vi "CheckStatusFlag.vi"(8 "error in (no error)":errorcluster, 11 "CS++Message in":refnum<class "CS++Message.lvclass">) -> (0 "error out":errorcluster, 3 "CS++Message out":refnum<class "CS++Message.lvclass">)   [LabVIEW 2016, in "CS++Message.lvlib" / "CS++Message.lvclass"]
uses:
  CS++Message.lvclass
  CS++Message.lvclass/CS++Message.ctl
  MessageStatus.ctl
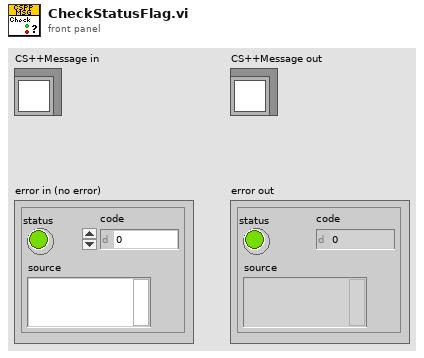
[diagram p1: front panel]
types:
  T1 = typedef "CS++Message.lvlib/CS++Message.lvclass/MessageStatus.ctl" = u16
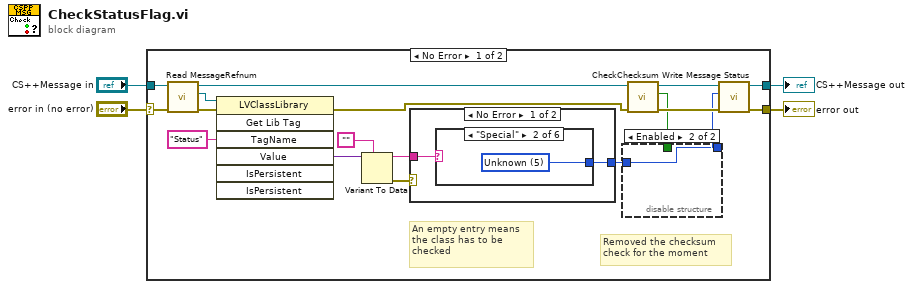
[diagram p0: block diagram]
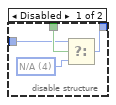
[diagram p2: hidden frame]
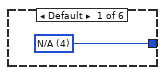
[diagram p3: hidden frame]
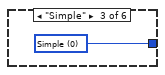
[diagram p4: hidden frame]
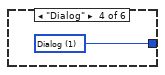
[diagram p5: hidden frame]
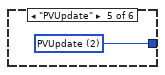
[diagram p6: hidden frame]
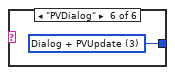
[diagram p7: hidden frame]
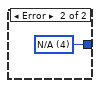
[diagram p8: hidden frame]
diagram:
  n1 = case shown="No Error" "error in (no error)" {
    selector: "error in (no error)" -> [w16 w38]
    tunnel: [w9 w38] -> w3
    tunnel: [w10 w37] -> w1
    tunnel: "CS++Message in" -> [w17 w37]
    frame No Error {
      # "Removed the checksum\ncheck for the moment"
      # "An empty entry means\nthe class has to be \nchecked"
      n2 = call "Read MessageRefnum.vi"("error in (no error)"=w16, "CS++Message in"=w17) -> ("error out"=w15:errorcluster, "MessageRefnum"=w14:refnum<vi>, "CS++Message out"=w13:refnum<class "CS++Message.lvclass">)  [unwired: 7 in]
      n3 = invoke class="LVClassLibrary" method="Get Lib Tag"(reference=w14, error in=w15, "TagName"="Status" ("Tag Name")) -> (error out=w12:errorcluster, "Value"=w21:variant)  [unwired: 4 in, 5 out]
      n4 = Variant To Data(type="", Variant=w21) -> (data=w18:string, error out=w19:errorcluster)  [unwired: 1 in]
      n5 = case shown="No Error" w19 {
        tunnel: w18 -> [w29 _]
        tunnel: [w28 w36] -> w6
        frame No Error {
          n6 = case shown="\"Special\"" w29 {
            tunnel: [w30 w31 w32 w33 w34 w35] -> w28
            frame Default {
              w30 = T1 4 items=["Simple", "Dialog", "PVUpdate", "Dialog + PVUpdate", "N/A"] ("Message Status")
            }
            frame "Special" {
              w31 = T1 5 items=["Simple", "Dialog", "PVUpdate", "Dialog + PVUpdate", "N/A", "Unknown"] ("Message Status")
            }
            frame "Simple" {
              w32 = T1 0 items=["Simple", "Dialog", "PVUpdate", "Dialog + PVUpdate", "N/A"] ("Message Status")
            }
            frame "Dialog" {
              w33 = T1 1 items=["Simple", "Dialog", "PVUpdate", "Dialog + PVUpdate", "N/A"] ("Message Status")
            }
            frame "PVUpdate" {
              w34 = T1 2 items=["Simple", "Dialog", "PVUpdate", "Dialog + PVUpdate", "N/A"] ("Message Status")
            }
            frame "PVDialog" {
              w35 = T1 3 items=["Simple", "Dialog", "PVUpdate", "Dialog + PVUpdate", "N/A"] ("Message Status")
            }
          }
        }
        frame Error {
          w36 = T1 4 items=["Simple", "Dialog", "PVUpdate", "Dialog + PVUpdate", "N/A"] ("Message Status")
        }
      }
      n7 = call "CheckChecksum.vi"("error in (no error)"=w12, "CS++Message in"=w13) -> ("error out"=w8:errorcluster, "ok?"=w7:bool, "CS++Message out"=w11:refnum<class "CS++Message.lvclass">)  [unwired: 7 in]
      n8 = disable-structure shown="Enabled" {
        disable-tunnel: w7 -> [w26 _]
        disable-tunnel: w6 -> [w25 w27]
        disable-tunnel: [w24 w27] -> w5
        frame Disabled {
          w23 = T1 4 items=["Simple", "Dialog", "PVUpdate", "Dialog + PVUpdate", "N/A"] ("Message Status")
          n9 = Select(t=w25, s=w26, f=w23) -> (s? t:f=w24:T1)
        }
        frame Enabled {
        }
      }
      n10 = call "Write Message Status.vi"("error in (no error)"=w8, "Message Status"=w5, "CS++Message in"=w11) -> ("error out"=w9:errorcluster, "CS++Message out"=w10:refnum<class "CS++Message.lvclass">)  [unwired: 7 in]
    }
    frame Error {
    }
  }
  "error out" <- w3
  "CS++Message out" <- w1
